vi "Error Query.vi"(8 "error in (no error)":errorcluster, 11 "VISA resource name":refnum<visa-resource-name>) -> (0 "error out":errorcluster, 1 "Error Message":string, 2 "Error Code":i32[](array[numeric]), 3 "VISA resource name out":refnum<visa-resource-name>)   [LabVIEW 2018, in "Keithley 24XX.lvlib"]
doc: "Queries the instrument for any errors in the instrument's error queue. It will continue to read errors until all errors have been read from the instrument. Any errors will be returned in the <B>error out</B> control.\n\nNote:\nThis VI is called automatically by most driver VIs so it is not usually necessary to call this in an application."
uses:
  Keithley 24XX.lvlib
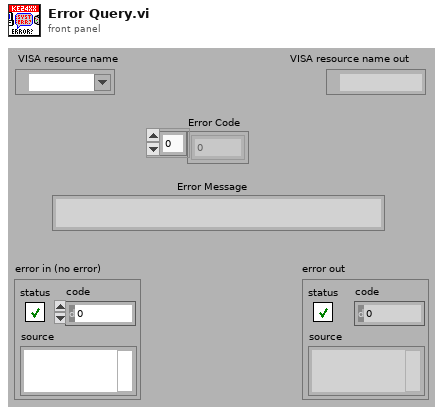
[diagram p1: front panel]
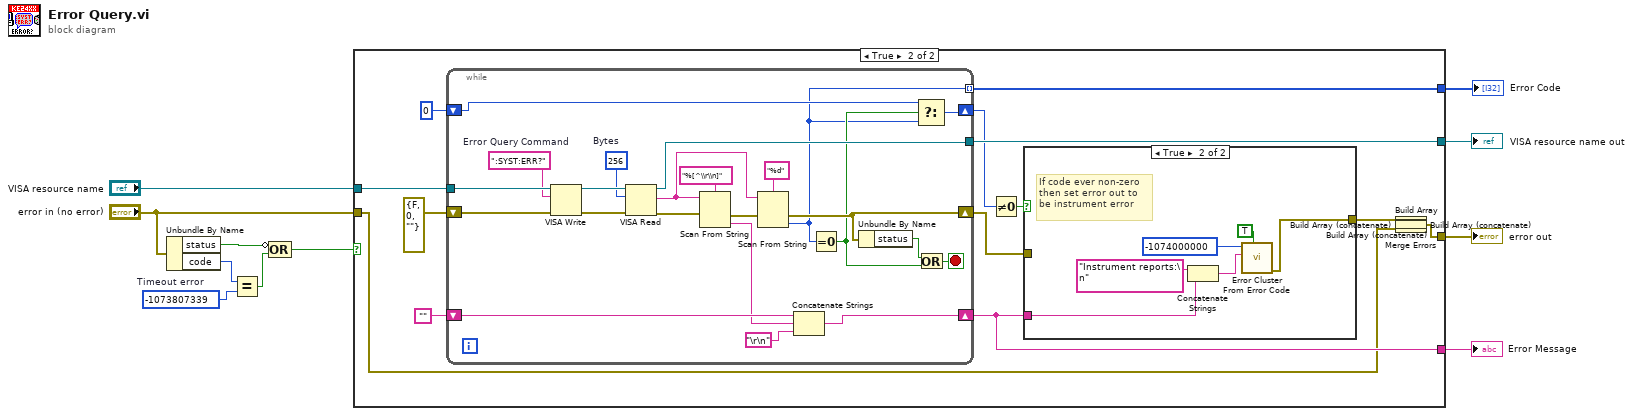
[diagram p0: block diagram]
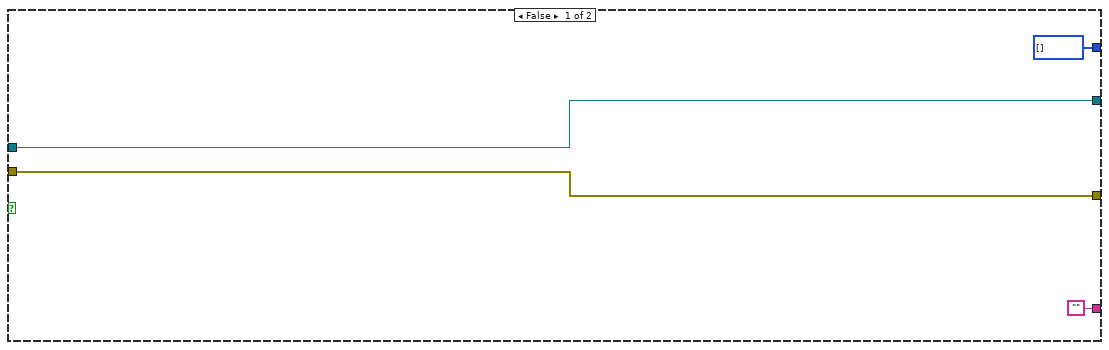
[diagram p2: hidden frame]
diagram:
  w6 = -1073807339  # Timeout error
  n1 = Unbundle By Name("error in (no error)") -> ("status"=w7:bool, "code"=w4:i32)
  n2 = Equal?(x=w4, y=w6) -> (x = y?=w5:bool)
  n3 = Compound Arithmetic op=OR(invert w7, w5) -> (w3:bool)
  n4 = case shown="True" w3 {
    tunnel: [w15 w32] -> w11
    tunnel: "VISA resource name" -> [w15 w31]
    tunnel: "error in (no error)" -> [w14 w21]
    tunnel: [w14 w29] -> w9
    tunnel: ["" w23] -> w2
    tunnel: [i32[] [] w22] -> w1
    frame False {
    }
    frame True {
      n5 = while {
        tunnel: [w62] -> w32
        tunnel: w31 -> [w61]
        shift-right: [w49] -> w23
        shift-left: "" -> [w52]
        shift-right: [w47] -> w24
        shift-left: 0 -> [w48]
        shift-right: [w45] -> w20
        shift-left: errorcluster {"status"=FALSE, "code"=0, "source"=""} ("error in (no error)") -> [w46]
        tunnel: [w40] -> w22 mode=indexing
        stop <- w55 stop-if-true
        w59 = u32 256  # Bytes
        w57 = ":SYST:ERR?"  # Error Query Command
        n6 = VISA Write(VISA resource name=w61, write buffer=w57, error in (no error)=w46) -> (VISA resource name out=w60:refnum<visa-resource-name>, error out=w58:errorcluster)  [unwired: 1 out]
        n7 = VISA Read(VISA resource name=w60, byte count=w59, error in (no error)=w58) -> (VISA resource name out=w62:refnum<visa-resource-name>, read buffer=w53:string, error out=w44:errorcluster)  [unwired: 1 out]
        n8 = Scan From String(format string="%[^\\r\\n]", input string=w53, error in=w44) -> (error out=w43:errorcluster, output 1=w50:string)  [unwired: 2 in, 2 out]
        n9 = Scan From String(format string="%d", input string=w53, error in=w43) -> (error out=w45:errorcluster, output 1=w40:i32)  [unwired: 2 in, 2 out]
        n10 = Concatenate Strings(w52, w50, "\r\n") -> (w49:string)
        n11 = Equal To 0?(x=w40) -> (x = 0?=w41:bool)
        n12 = Unbundle By Name(w45) -> ("status"=w42:bool)
        n13 = Select(t=w48, s=w41, f=w40) -> (s? t:f=w47:i32)
        n14 = Or(x=w42, y=w41) -> (x .or. y?=w55:bool)
      }
      n15 = Not Equal To 0?(x=w24) -> (x != 0?=w27:bool)
      n16 = case shown="True" w27 {
        tunnel: w23 -> [_ w38]
        tunnel: [w33 w34] -> w26
        tunnel: w20 -> [w33 _]
        frame False {
        }
        frame True {
          # "If code ever non-zero\nthen set error out to\nbe instrument error"
          n17 = Concatenate Strings("Instrument reports:\n" ("Source"), w38) -> (w35:string)
          n18 = call <vilib>:"Error Cluster From Error Code.vi"("show call chain? (False)"=TRUE, "error message (\"\")"=w35, "error code (0)"=-1074000000 ("Code")) -> ("error out"=w34:errorcluster)  [unwired: 6 in]
        }
      }
      n19 = Build Array(w26, w21) -> (w19:errorcluster[])
      n20 = Build Array (concatenate)(w19) -> (w18:errorcluster[])
      n21 = Build Array (concatenate)(w18) -> (w17:errorcluster[])
      n22 = Build Array (concatenate)(w17) -> (w16:errorcluster[])
      n23 = Merge Errors(w16) -> (w29:errorcluster)
    }
  }
  "VISA resource name out" <- w11
  "error out" <- w9
  "Error Message" <- w2
  "Error Code" <- w1
